vi "Decimate (2D).vi"(9 "averaging":bool, 10 "decimating factor":i32=1, 11 "X":dbl[][](array[numeric])) -> (0 "error":i32, 3 "Decimated Array":dbl[][](array[numeric]))   [LabVIEW 2015]
uses:
  <vilib>/Analysis/2dsp.llb/Decimate (single shot, DBL).vi
  <vilib>/Analysis/NI_AALPro.lvlib
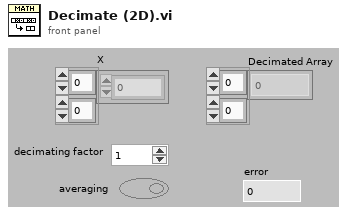
[diagram p1: front panel]
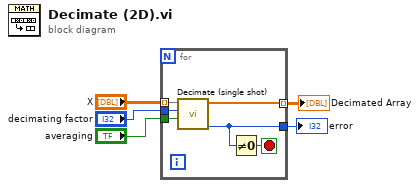
[diagram p0: block diagram]
diagram:
  n1 = for {
    tunnel: "X" -> [w11] mode=indexing
    tunnel: "decimating factor" -> [w10]
    tunnel: "averaging" -> [w9]
    tunnel: [w8] -> w2 mode=indexing
    tunnel: [w6] -> w1
    stop <- w7 stop-if-true
    n2 = call-poly <vilib>:"Decimate (single shot).vi"("averaging"=w9, "decimating factor"=w10, "X"=w11) -> ("error"=w6:i32, "Decimated Array"=w8:dbl[])  [unwired: 7 in]
    n3 = Not Equal To 0?(x=w6) -> (x != 0?=w7:bool)
  }
  "Decimated Array" <- w2
  "error" <- w1
